vi "Initialize-link.vi"(8 "error in (no error)":errorcluster, 11 "Motor-DAQmx in":refnum<class "Motor-DAQmx.lvclass">) -> (0 "error out":errorcluster, 3 "Motor-DAQmx out":refnum<class "Motor-DAQmx.lvclass">)   [LabVIEW 2013, in "PowderDeposition.lvlib" / "Motor-DAQmx.lvclass"]
uses:
  Motor-DAQmx.lvclass
  Motor-Analog.lvclass/Motor-Analog.ctl
  Motor-DAQmx.lvclass/Motor-DAQmx.ctl
  <vilib>/DAQmx/write.llb/DAQmx Write (Digital Bool 1Line 1Point).vi
  <vilib>/DAQmx/create/channels.llb/DAQmx Create Channel (DO-Digital Output).vi
  <vilib>/DAQmx/miscellaneous.llb/DAQmx Fill In Error Info.vi
  Motor-Analog.lvclass
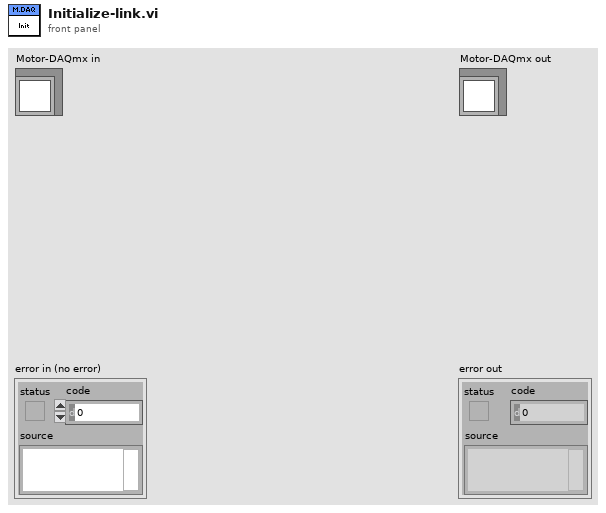
[diagram p1: front panel]
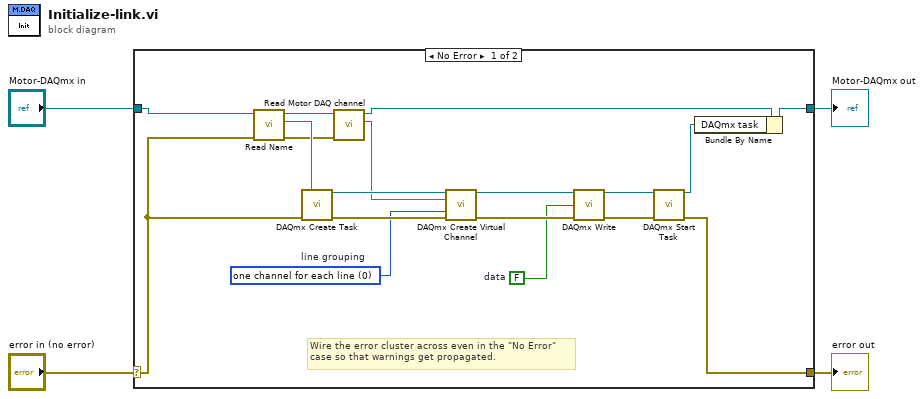
[diagram p0: block diagram]
diagram:
  n1 = case shown="No Error" "error in (no error)" {
    selector: "error in (no error)" -> [w18 w24]
    tunnel: [w5 w24] -> w3
    tunnel: [w12 w23] -> w1
    tunnel: "Motor-DAQmx in" -> [w17 w23]
    frame No Error {
      w7 = FALSE  # data
      w13 = 0 items=["one channel for each line", "one channel for all lines"]  # line grouping
      # "Wire the error cluster across even in the \"No Error\"\ncase so that warnings get propagated."
      n2 = call-dynamic "Read Name.vi"("error in (no error)"=w18, "Motor in"=w17) -> ("error out"=w19:errorcluster, "Name"=w21:string, "Motor out"=w20:refnum<class "Motor-DAQmx.lvclass">)  [unwired: 7 in]
      n3 = call <vilib>:"DAQmx Create Task.vi"("new task name"=w21, "error in"=w18) -> ("task out"=w16:refnum<k21>, "error out"=w22:errorcluster)  [unwired: 12 in]
      n4 = call "Read Motor DAQ channel.vi"("error in (no error)"=w19, "Motor-Analog in"=w20) -> ("Motor DAQ channel"=w14:tag, "Motor-Analog out"=w15:refnum<class "Motor-DAQmx.lvclass">)  [unwired: 7 in, 1 out]
      n5 = call-poly <vilib>:"DAQmx Create Virtual Channel.vi"("task in"=w16, "lines"=w14, "line grouping"=w13, "error in"=w22) -> ("task out"=w11:refnum<k21>, "error out"=w8:errorcluster)  [unwired: 10 in]
      n6 = call-poly <vilib>:"DAQmx Write.vi"("task/channels in"=w11, "data"=w7, "error in"=w8) -> ("task out"=w10:refnum<k21>, "error out"=w9:errorcluster)  [unwired: 10 in, 1 out]
      n7 = call <vilib>:"DAQmx Start Task.vi"("task/channels in"=w10, "error in"=w9) -> ("task out"=w6:refnum<k21>, "error out"=w5:errorcluster)  [unwired: 12 in]
      n8 = Bundle By Name(cluster=w15, "DAQmx task"=w6) -> (w12:refnum<class "Motor-DAQmx.lvclass">)
    }
    frame Error {
    }
  }
  "error out" <- w3
  "Motor-DAQmx out" <- w1
